vi "Disp.vi"(3 "Slot_color":enum16{"0", "1", "2"}(ring), 4 "index":i32, 5 "Slot":refnum<vi>[](array[refnum])) -> ()   [LabVIEW 8.6]
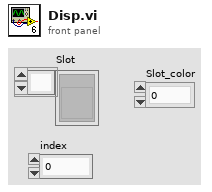
[diagram p1: front panel]
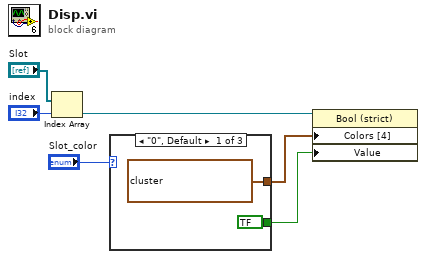
[diagram p0: block diagram]
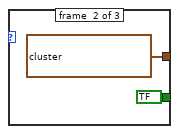
[diagram p2: hidden frame]
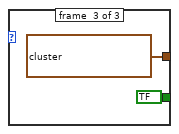
[diagram p3: hidden frame]
diagram:
  n1 = Index Array(array="Slot", index="index") -> (element=w1:refnum<vi>)
  n2 = case shown="\"0\", Default" "Slot_color" {
    tunnel: [bool ? bool ? bool ?] -> w4
    tunnel: [cluster{u32, u32}[] ? ("Colors [4]") cluster{u32, u32}[] ? ("Colors [4]") cluster{u32, u32}[] ? ("Colors [4]")] -> w5
    frame #0 {
    }
    frame #1 {
    }
    frame #2 {
    }
  }
  n3 = property on="Property Node" class="Bool (strict)"(reference=w1, "Colors [4]"=w5, "Value"=w4) -> ()  [unwired: 1 in, 2 out]
